vi "Icon Editor Init Refs.vi"(8 "error in (no error)":errorcluster, 10 "Ref Cluster":T1) -> (0 "error out":errorcluster)   [LabVIEW 2021]
uses:
  <resource>/plugins/NIIconEditor/Controls/References Cluster.ctl
  <vilib>/LabVIEW Icon API/lv_icon/Controls/Layer.ctl
  <vilib>/LabVIEW Icon API/lv_icon/lv_icon.lvlib
panel:
  in  "Localized tag":string="Import Icon from Owning Library"
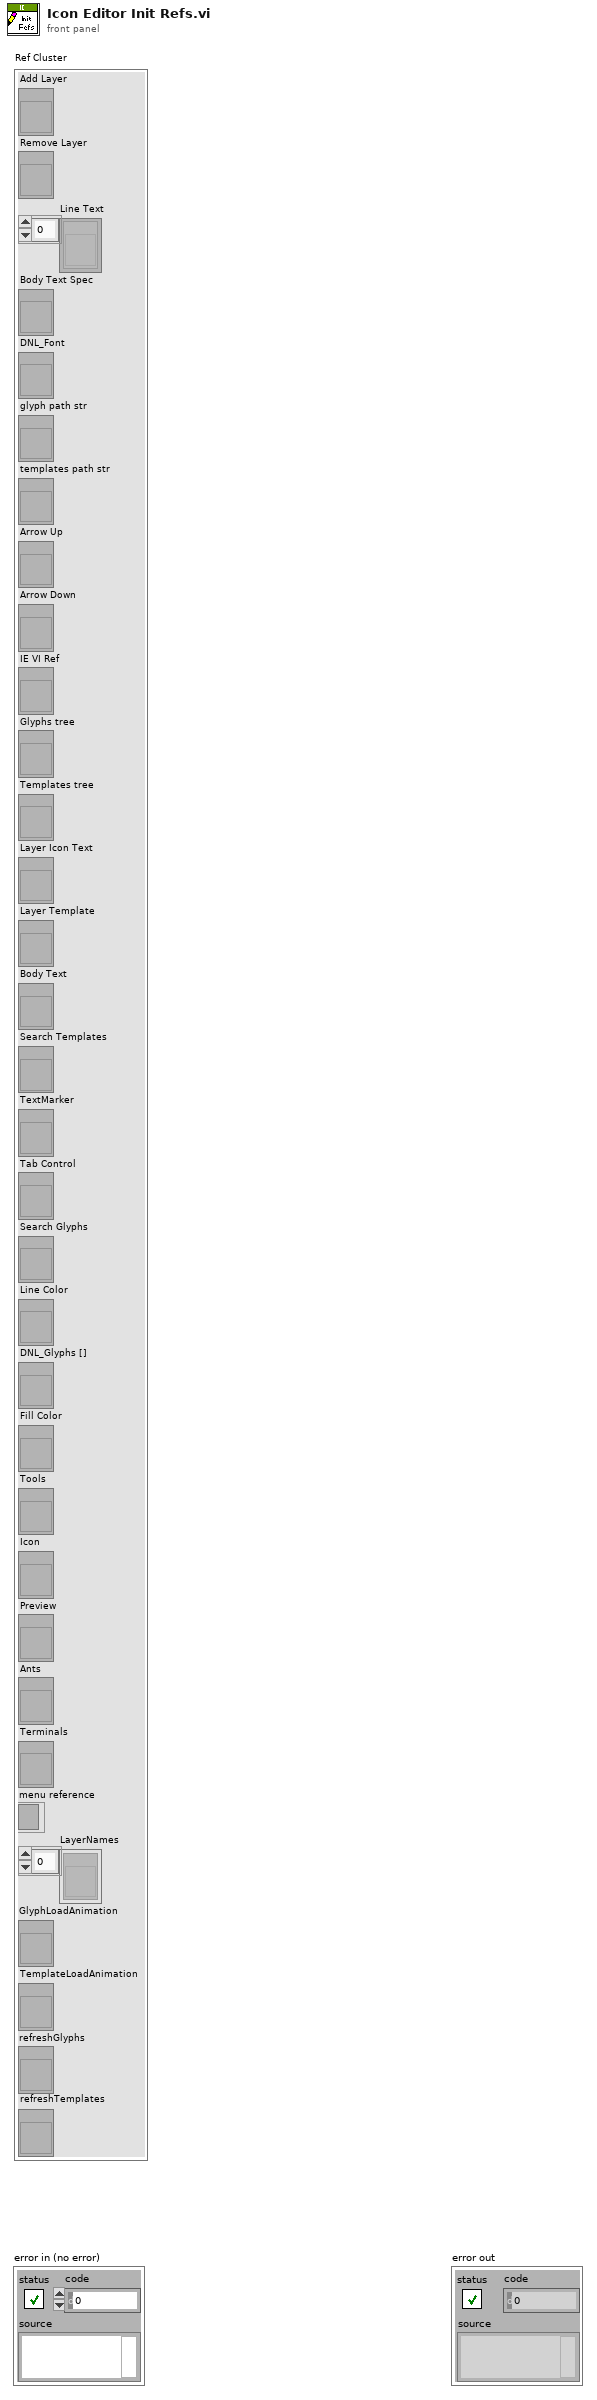
[diagram p1: front panel]
types:
  T1 = typedef "lv_icon.lvlib/References Cluster.ctl" = cluster{"Add Layer":refnum<vi>, "Remove Layer":refnum<vi>, "Line Text":refnum<vi>[], "Body Text Spec":refnum<vi>, "DNL_Font":refnum<vi>, "glyph path str":refnum<vi>, "templates path str":refnum<vi>, "Arrow Up":refnum<vi>, "Arrow Down":refnum<vi>, "IE VI Ref":refnum<vi>, "Glyphs tree":refnum<vi>, "Templates tree":refnum<vi>, "Layer Icon Text":refnum<vi>, "Layer Template":refnum<vi>, "Body Text":refnum<vi>, "Search Templates":refnum<vi>, "TextMarker":refnum<vi>, "Tab Control":refnum<vi>, "Search Glyphs":refnum<vi>, "Line Color":refnum<vi>, "DNL_Glyphs []":refnum<vi>, "Fill Color":refnum<vi>, "Tools":refnum<vi>, "Icon":refnum<vi>, "Preview":refnum<vi>, "Ants":refnum<vi>, "Terminals":refnum<vi>, "menu reference":refnum<k9>, "LayerNames":refnum<vi>[], "GlyphLoadAnimation":refnum<vi>, "TemplateLoadAnimation":refnum<vi>, "refreshGlyphs":refnum<vi>, "refreshTemplates":refnum<vi>}
  T2 = typedef "Layer.ctl" = cluster{"LayerIcon":picture, "LayerName":string, "Opacity":u8, "Visibility?":bool}
  T3 = typedef "lv_icon.lvlib/INI Data.ctl" = cluster{"Show Terminals?":bool, "Text":cluster{"Font":T4, "Alignment":T5, "Size":T6}, "3rd party Templates":cluster{"Store 3rd party Templates?":bool, "Folder Name":string}, "Merge user layers on commit":bool, "Body Text":T7, "Fill Color":T8, "Edge Color":T8, "Tab":u16, "Tool":T9, "Disable Layers?":bool}
  T4 = typedef "Font.ctl" = string
  T5 = typedef "Alignment.ctl" = u16
  T6 = typedef "Font Size.ctl" = u8
  T7 = typedef "BodyText.ctl" = cluster{"Line 1 text":string, "Line 2 text":string, "Line 3 text":string, "Line 4 text":string, "Line 1 color":u32, "Line 2 color":u32, "Line 3 color":u32, "Line 4 color":u32, "Body Text Spec":cluster{"Font":T4, "Alignment":T5, "Size":u8}, "Center text vertically":bool, "Capitalize Text":bool}
  T8 = typedef "IEColor.ctl" = u32
  T9 = typedef "Tools.ctl" = enum32{"Pencil", "Line", "Dropper", "Fill", "Rectangle", "Filled Rectangle", "Ellipse", "Filled Ellipse", "Eraser", "Text", "Select", "Move"}
  T10 = typedef "LabVIEW Icon Stored Information.ctl" = cluster{"Text Visible?":bool, "Text Opacity":u8, "Templ Visible?":bool, "Templ Opacity":u8, "Relative Path from 1 to 2":path, "Image":picture, "All User Layers":refnum<class "Layer.lvclass">[], "Body Text":T7}
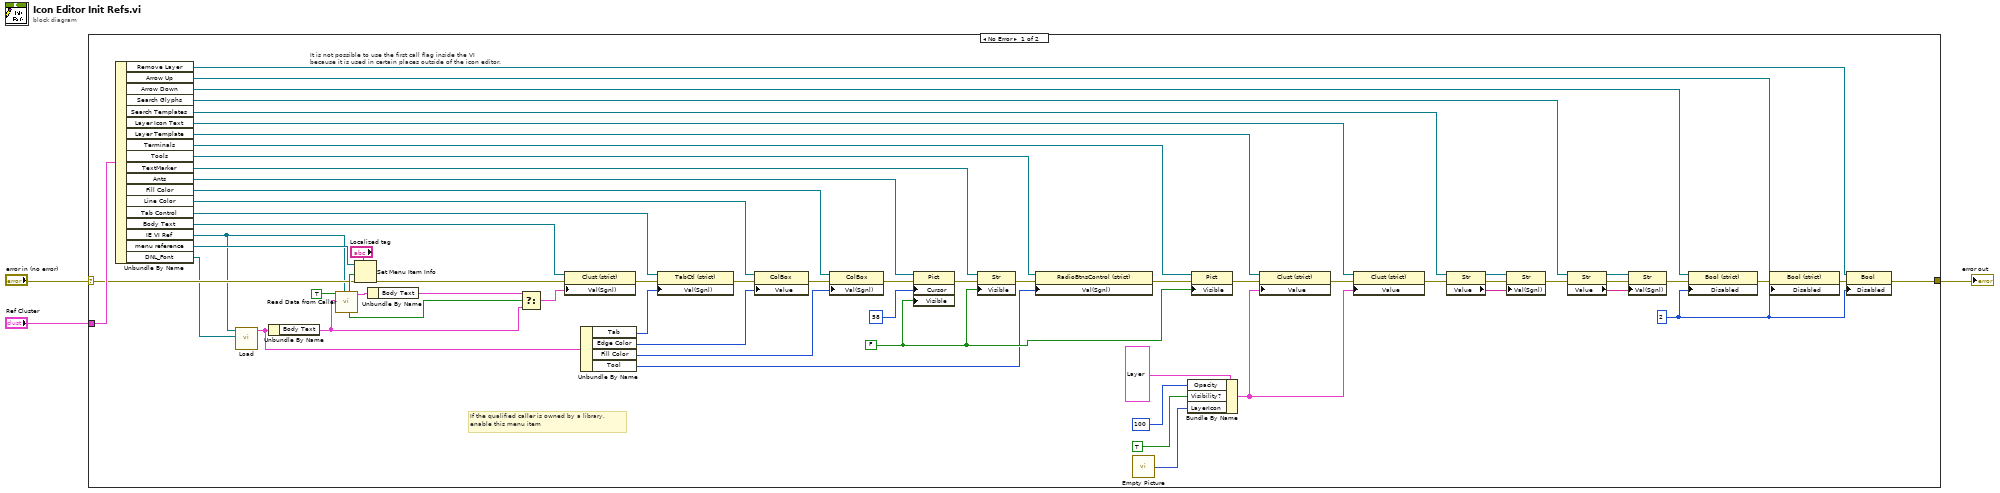
[diagram p0: block diagram]
diagram:
  n1 = case shown="No Error" "error in (no error)" {
    selector: "error in (no error)" -> [w9 w67]
    tunnel: [w15 w67] -> w2
    tunnel: "Ref Cluster" -> [w40 _]
    frame No Error {
      w14 = u8 2 ("Disabled")
      w49 = FALSE ("Visible")
      # "If the qualified caller is owned by a library,\nenable this menu item"
      # "It is not possible to use the first call flag inside the VI\nbecause it is used in certain places outside of the icon editor."
      n2 = Unbundle By Name(w40) -> ("Remove Layer"=w13:refnum<vi>, "Arrow Up"=w38:refnum<vi>, "Arrow Down"=w39:refnum<vi>, "Search Glyphs"=w29:refnum<vi>, "Search Templates"=w36:refnum<vi>, "Layer Icon Text"=w22:refnum<vi>, "Layer Template"=w41:refnum<vi>, "Terminals"=w51:refnum<vi>, "Tools"=w54:refnum<vi>, "TextMarker"=w55:refnum<vi>, "Ants"=w57:refnum<vi>, "Fill Color"=w65:refnum<vi>, "Line Color"=w66:refnum<vi>, "Tab Control"=w48:refnum<vi>, "Body Text"=w19:refnum<vi>, "IE VI Ref"=w5:refnum<vi>, "menu reference"=w10:refnum<k9>, "DNL_Font"=w4:refnum<vi>)
      n3 = call <resource>:"Load.vi"("DNL_Font"=w4, "IE VI Ref"=w5) -> ("INI Data"=w7:T3)  [unwired: 1 in, 8 out]
      n4 = Unbundle By Name(w7) -> ("Body Text"=w6:T7)
      n5 = call <resource>:"Read Data from Caller.vi"("lv_icon.vi"=w5, "Default body text"=w6, "Init? (F)"=TRUE) -> ("data"=w60:T10, "Valid?"=w61:bool, "Valid Library icon?"=w11:bool)  [unwired: 1 in, 5 out]
      n6 = Set Menu Item Info(7:"Localized tag", 8:w9, 9:w11, 11:w10) -> (0:w8:errorcluster)  [unwired: 3 in, 1 out]
      n7 = Unbundle By Name(w60) -> ("Body Text"=w59:T7)
      n8 = Select(t=w59, s=w61, f=w6) -> (s? t:f=w58:T7)
      n9 = property class="Clust (strict)"(reference=w19, error in=w8, "Val(Sgnl)"=w58) -> (error out=w18:errorcluster)  [unwired: 1 out]
      n10 = Unbundle By Name(w7) -> ("Tab"=w46:u16, "Edge Color"=w63:T8, "Fill Color"=w62:T8, "Tool"=w45:T9)
      n11 = property class="TabCtl (strict)"(reference=w48, error in=w18, "Val(Sgnl)"=w46) -> (error out=w47:errorcluster)  [unwired: 1 out]
      n12 = property class="ColBox"(reference=w66, error in=w47, "Value"=w63) -> (error out=w64:errorcluster)  [unwired: 1 out]
      n13 = property class="ColBox"(reference=w65, error in=w64, "Val(Sgnl)"=w62) -> (error out=w17:errorcluster)  [unwired: 1 out]
      n14 = property class="Pict"(reference=w57, error in=w17, "Cursor"=58, "Visible"=w49) -> (error out=w53:errorcluster)  [unwired: 1 out]
      n15 = property class="Str"(reference=w55, error in=w53, "Visible"=w49) -> (error out=w52:errorcluster)  [unwired: 1 out]
      n16 = property class="RadioBtnsControl (strict)"(reference=w54, error in=w52, "Val(Sgnl)"=w45) -> (error out=w50:errorcluster)  [unwired: 1 out]
      n17 = call "Empty Picture"() -> ("empty picture"=w43:picture)
      n18 = Bundle By Name(cluster=T2 {"LayerIcon"=bytes[0], "LayerName"="", "Opacity"=0, "Visibility?"=FALSE} ("Value (Signaling)"), "Opacity"=u8 100, "Visibility?"=TRUE, "LayerIcon"=w43) -> (w21:T2)
      n19 = property class="Pict"(reference=w51, error in=w50, "Visible"=w49) -> (error out=w42:errorcluster)  [unwired: 1 out]
      n20 = property class="Clust (strict)"(reference=w41, error in=w42, "Value"=w21) -> (error out=w23:errorcluster)  [unwired: 1 out]
      n21 = property class="Clust (strict)"(reference=w22, error in=w23, "Value"=w21) -> (error out=w20:errorcluster)  [unwired: 1 out]
      n22 = property class="Str"(reference=w36, error in=w20) -> (reference out=w35:refnum<vi>, error out=w34:errorcluster, "Value"=w33:string)
      n23 = property class="Str"(reference=w35, error in=w34, "Val(Sgnl)"=w33) -> (error out=w28:errorcluster)  [unwired: 1 out]
      n24 = property class="Str"(reference=w29, error in=w28) -> (reference out=w30:refnum<vi>, error out=w31:errorcluster, "Value"=w32:string)
      n25 = property class="Str"(reference=w30, error in=w31, "Val(Sgnl)"=w32) -> (error out=w27:errorcluster)  [unwired: 1 out]
      n26 = property class="Bool (strict)"(reference=w39, error in=w27, "Disabled"=w14) -> (error out=w37:errorcluster)  [unwired: 1 out]
      n27 = property class="Bool (strict)"(reference=w38, error in=w37, "Disabled"=w14) -> (error out=w16:errorcluster)  [unwired: 1 out]
      n28 = property class="Bool"(reference=w13, error in=w16, "Disabled"=w14) -> (error out=w15:errorcluster)  [unwired: 1 out]
    }
    frame Error {
    }
  }
  "error out" <- w2
